vi "TDMS_Channel_Initialize.vi"(9 "Channel":string, 10 "Group":string, 11 "TDMS":string) -> (3 "TDMS Channel Info":T1)   [LabVIEW 2015]
uses:
  <userlib>/836-Library/System/TDMSv2/TDMS_Channel_Info.ctl
  <userlib>/836-Library/System/TDMSv2/TDMS_RT_FIFO_Packet.ctl
  <userlib>/836-Library/System/TDMSv2/Back_Channel_Data.ctl
  <userlib>/836-Library/System/TDMSv2/GroupChannelIDs.ctl
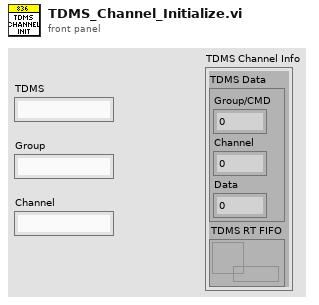
[diagram p1: front panel]
types:
  T1 = typedef "TDMS_Channel_Info.ctl" = cluster{"TDMS Data":T2, "TDMS RT FIFO":refnum<k33>}
  T2 = typedef "TDMS_RT_FIFO_Packet.ctl" = cluster{"Group/CMD":i32, "Channel":i32, "Data":dbl}
  T3 = cluster{"TDMS Data":T2, "TDMS RT FIFO":refnum<k33>}
  T4 = typedef "GroupChannelIDs.ctl" = cluster{"Group":i32, "Channel":i32}
  T5 = typedef "Back_Channel_Data.ctl" = cluster{"Group":string, "Channel":string, "Return Notifier":refnum<notifier>}
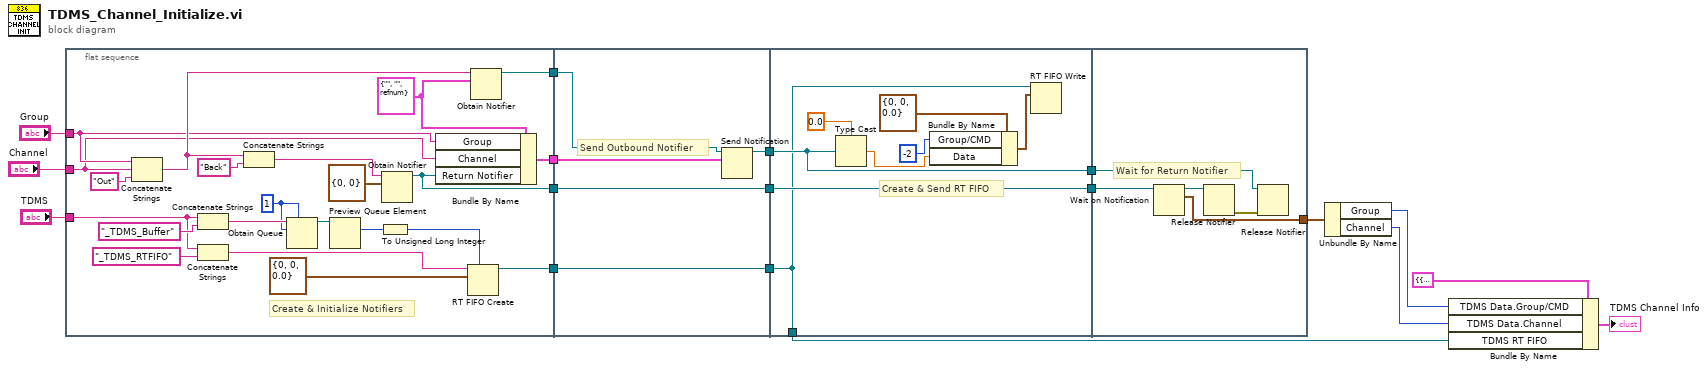
[diagram p0: block diagram]
diagram:
  n1 = flat-sequence {
    tunnel: "Group" -> [w36]
    tunnel: "Channel" -> [w35]
    tunnel: [w34] -> w18
    tunnel: [w32] -> w17
    tunnel: [w30] -> w16
    tunnel: [w29] -> w15
    tunnel: "TDMS" -> [w23]
    tunnel: w18 -> [w45]
    tunnel: [w44] -> w14
    tunnel: w17 -> [w44]
    tunnel: [w43] -> w13
    tunnel: w16 -> [w42]
    tunnel: [w41] -> w12
    tunnel: w15 -> [w41]
    tunnel: [w52] -> w11
    tunnel: w14 -> [w52]
    tunnel: [w51] -> w10
    tunnel: w13 -> [w51]
    tunnel: w12 -> [w46]
    tunnel: [w46] -> w2
    tunnel: w11 -> [w58]
    tunnel: w10 -> [w55]
    tunnel: [w54] -> w6
    frame #0 {
      w22 = 1 ("max queue size (-1, unlimited)")
      w31 = T5 {"Group"="", "Channel"="", "Return Notifier"=refnum}
      # "Create & Initialize Notifiers"
      n2 = Concatenate Strings(w36, w35, "Out" ("string")) -> (w40:string)
      n3 = Concatenate Strings(w23, "_TDMS_Buffer" ("string")) -> (w25:string)
      n4 = Concatenate Strings(w23, "_TDMS_RTFIFO" ("string")) -> (w27:string)
      n5 = Concatenate Strings(w40, "Back" ("string")) -> (w39:string)
      n6 = Obtain Queue(max queue size (-1, unlimited)=w22, name (unnamed)=w25, element data type=w22) -> (queue out=w21:refnum<queue>)  [unwired: 2 in, 2 out]
      n7 = Preview Queue Element(queue=w21) -> (element=w20:i32)  [unwired: 2 in, 3 out]
      n8 = To Unsigned Long Integer(number=w20) -> (unsigned 32bit integer=w19:u32)
      n9 = Obtain Notifier(name (unnamed)=w39, notification data type=T4 {"Group"=0, "Channel"=0}) -> (notifier out=w32:refnum<notifier>)  [unwired: 2 in, 2 out]
      n10 = Bundle By Name(cluster=w31, "Group"=w36, "Channel"=w35, "Return Notifier"=w32) -> (w30:T5)
      n11 = RT FIFO Create(0:w27, 1:T2 {"Group/CMD"=0, "Channel"=0, "Data"=0.0}, 4:w19) -> (8:w29:refnum<k33>)  [unwired: 5 in, 2 out]
      n12 = Obtain Notifier(name (unnamed)=w40, notification data type=w31) -> (notifier out=w34:refnum<notifier>)  [unwired: 2 in, 2 out]
    }
    frame #1 {
      # "Send Outbound Notifier"
      n13 = Send Notification(notification=w42, notifier=w45) -> (notifier out=w43:refnum<notifier>)  [unwired: 1 in, 1 out]
    }
    frame #2 {
      # "Create & Send RT FIFO"
      n14 = Type Cast(type=0.0, x=w51) -> (*(type *) &x=w49:dbl)
      n15 = Bundle By Name(cluster=T2 {"Group/CMD"=0, "Channel"=0, "Data"=0.0}, "Group/CMD"=-2, "Data"=w49) -> (w47:T2)
      n16 = RT FIFO Write(0:w46, 1:w47) -> ()  [unwired: 3 in, 4 out]
    }
    frame #3 {
      # "Wait for Return Notifier"
      n17 = Wait on Notification(notifier=w58) -> (notifier out=w57:refnum<notifier>, notification=w54:T4)  [unwired: 3 in, 2 out]
      n18 = Release Notifier(notifier=w57) -> (error out=w56:errorcluster)  [unwired: 2 in, 2 out]
      n19 = Release Notifier(notifier=w55, error in (no error)=w56) -> ()  [unwired: 1 in, 3 out]
    }
  }
  n20 = Unbundle By Name(w6) -> ("Group"=w5:i32, "Channel"=w4:i32)
  n21 = Bundle By Name(cluster=T3 {"TDMS Data"={"Group/CMD"=0, "Channel"=0, "Data"=0.0}, "TDMS RT FIFO"=refnum}, "TDMS Data.Group/CMD"=w5, "TDMS Data.Channel"=w4, "TDMS RT FIFO"=w2) -> (→"TDMS Channel Info":T3)
